vi "HelloWorld.vi"   [LabVIEW 2026]
uses:
  SDL3/Video/WindowFlags--ring.ctl
  SDL3/Pixels/PixelFormat--enum.ctl
  SDL3/Render/TextureAccess-enum.ctl
  SDL3/Init/InitFlags--ring.ctl
  SDL3/Events/MouseMotionEvent--cluster.ctl
  SDL3/Video/WindowID--integer.ctl
  SDL3/Mouse/MouseID--integer.ctl
  SDL3/Mouse/MouseButtonFlags--ring.ctl
  SDL3/Rect/FRect--cluster.ctl
  SDL3/Error/GetError-UiThread.vi
  SDL3/Error/GetError-AnyThread.vi
  SDL3/Pixels/PixelFormatEnumToU32.vi
  SDL3/LV-Utilities/IsNULL.vi
  SDL3/Pixels/U32ToPixelFormatEnum.vi
  <vilib>/Utility/error.llb/Error Cluster From Error Code.vi
  SDL3/Init/Init.lvlib
  SDL3/Video/Video.lvlib
  SDL3/Render/Render.lvlib
  SDL3/Pixels/Pixels.lvlib
  SDL3/Timer/Timer.lvlib
  SDL3/Events/Events.lvlib
  SDL3/Mouse/Mouse.lvlib
  SDL3/TTF/TTF.lvlib
  SDL3/Surface/Surface.lvlib
  SDL3/Rect/Rect.lvlib
types:
  T1 = enum32{"Invalid", "Standard", "Closed", "Hidden", "Minimized", "Maximized"}
  T2 = typedef "SDL3.lvlib/Events.lvlib/MouseMotionEvent--cluster.ctl" = cluster{"Timestamp":u64, "Window ID":T3, "Which":T4, "State":T5, "x":sgl, "y":sgl, "x Rel":sgl, "y Rel":sgl}
  T3 = typedef "SDL3.lvlib/Video.lvlib/WindowID--integer.ctl" = u32
  T4 = typedef "SDL3.lvlib/Mouse.lvlib/MouseID--integer.ctl" = u32
  T5 = typedef "SDL3.lvlib/Mouse.lvlib/MouseButtonFlags--ring.ctl" = u32
  T6 = typedef "SDL3.lvlib/Init.lvlib/InitFlags--ring.ctl" = u32
  T7 = typedef "SDL3.lvlib/Render.lvlib/TextureAccess-enum.ctl" = enum32{"SDL_TEXTUREACCESS_STATIC", "SDL_TEXTUREACCESS_STREAMING", "SDL_TEXTUREACCESS_TARGET"}
  T8 = typedef "SDL3.lvlib/Pixels.lvlib/PixelFormat--enum.ctl" = enum32{"SDL_PIXELFORMAT_UNKNOWN", "SDL_PIXELFORMAT_INDEX1LSB", "SDL_PIXELFORMAT_INDEX1MSB", "SDL_PIXELFORMAT_INDEX2LSB", "SDL_PIXELFORMAT_INDEX2MSB", "SDL_PIXELFORMAT_INDEX4LSB", "SDL_PIXELFORMAT_INDEX4MSB", "SDL_PIXELFORMAT_INDEX8", "SDL_PIXELFORMAT_RGB332", "SDL_PIXELFORMAT_XRGB4444", "SDL_PIXELFORMAT_XBGR4444", "SDL_PIXELFORMAT_XRGB1555", "SDL_PIXELFORMAT_XBGR1555", "SDL_PIXELFORMAT_ARGB4444", "SDL_PIXELFORMAT_RGBA4444", "SDL_PIXELFORMAT_ABGR4444", "SDL_PIXELFORMAT_BGRA4444", "SDL_PIXELFORMAT_ARGB1555", "SDL_PIXELFORMAT_RGBA5551", "SDL_PIXELFORMAT_ABGR1555", "SDL_PIXELFORMAT_BGRA5551", "SDL_PIXELFORMAT_RGB565", "SDL_PIXELFORMAT_BGR565", "SDL_PIXELFORMAT_RGB24", "SDL_PIXELFORMAT_BGR24", "SDL_PIXELFORMAT_XRGB8888", "SDL_PIXELFORMAT_RGBX8888", "SDL_PIXELFORMAT_XBGR8888", "SDL_PIXELFORMAT_BGRX8888", "SDL_PIXELFORMAT_ARGB8888", "SDL_PIXELFORMAT_RGBA8888", "SDL_PIXELFORMAT_ABGR8888", "SDL_PIXELFORMAT_BGRA8888", "SDL_PIXELFORMAT_XRGB2101010", "SDL_PIXELFORMAT_XBGR2101010", "SDL_PIXELFORMAT_ARGB2101010", "SDL_PIXELFORMAT_ABGR2101010", "SDL_PIXELFORMAT_RGB48", "SDL_PIXELFORMAT_BGR48", "SDL_PIXELFORMAT_RGBA64", "SDL_PIXELFORMAT_ARGB64", "SDL_PIXELFORMAT_BGRA64", "SDL_PIXELFORMAT_ABGR64", "SDL_PIXELFORMAT_RGB48_FLOAT", "SDL_PIXELFORMAT_BGR48_FLOAT", "SDL_PIXELFORMAT_RGBA64_FLOAT", "SDL_PIXELFORMAT_ARGB64_FLOAT", "SDL_PIXELFORMAT_BGRA64_FLOAT", "SDL_PIXELFORMAT_ABGR64_FLOAT", "SDL_PIXELFORMAT_RGB96_FLOAT", "SDL_PIXELFORMAT_BGR96_FLOAT", "SDL_PIXELFORMAT_RGBA128_FLOAT", "SDL_PIXELFORMAT_ARGB128_FLOAT", "SDL_PIXELFORMAT_BGRA128_FLOAT", "SDL_PIXELFORMAT_ABGR128_FLOAT", "SDL_PIXELFORMAT_YV12", "SDL_PIXELFORMAT_IYUV", "SDL_PIXELFORMAT_YUY2", "SDL_PIXELFORMAT_UYVY", "SDL_PIXELFORMAT_YVYU", "SDL_PIXELFORMAT_NV12", "SDL_PIXELFORMAT_NV21", "SDL_PIXELFORMAT_P010", "SDL_PIXELFORMAT_EXTERNAL_OES"}
  T9 = typedef "SDL3.lvlib/Video.lvlib/WindowFlags--ring.ctl" = u64
  T10 = typedef "SDL3.lvlib/Rect.lvlib/FRect--cluster.ctl" = cluster{"x":sgl, "y":sgl, "w":sgl, "h":sgl}
  T11 = typedef "SDL3.lvlib/Events.lvlib/EventType--enum.ctl" = enum16{"LV_NONE", "LV_UNSUPPORTED", "SDL_EVENT_QUIT", "SDL_EVENT_LOCALE_CHANGED", "SDL_EVENT_SYSTEM_THEME_CHANGED", "SDL_EVENT_DISPLAY_ORIENTATION", "SDL_EVENT_DISPLAY_ADDED", "SDL_EVENT_DISPLAY_REMOVED", "SDL_EVENT_DISPLAY_MOVED", "SDL_EVENT_DISPLAY_DESKTOP_MODE_CHANGED", "SDL_EVENT_DISPLAY_CURRENT_MODE_CHANGED", "SDL_EVENT_DISPLAY_CONTENT_SCALE_CHANGED", "SDL_EVENT_WINDOW_SHOWN", "SDL_EVENT_WINDOW_HIDDEN", "SDL_EVENT_WINDOW_EXPOSED", "SDL_EVENT_WINDOW_MOVED", "SDL_EVENT_WINDOW_RESIZED", "SDL_EVENT_WINDOW_PIXEL_SIZE_CHANGED", "SDL_EVENT_WINDOW_METAL_VIEW_RESIZED", "SDL_EVENT_WINDOW_MINIMIZED", "SDL_EVENT_WINDOW_MAXIMIZED", "SDL_EVENT_WINDOW_RESTORED", "SDL_EVENT_WINDOW_MOUSE_ENTER", "SDL_EVENT_WINDOW_MOUSE_LEAVE", "SDL_EVENT_WINDOW_FOCUS_GAINED", "SDL_EVENT_WINDOW_FOCUS_LOST", "SDL_EVENT_WINDOW_CLOSE_REQUESTED", "SDL_EVENT_WINDOW_HIT_TEST", "SDL_EVENT_WINDOW_ICCPROF_CHANGED", "SDL_EVENT_WINDOW_DISPLAY_CHANGED", "SDL_EVENT_WINDOW_DISPLAY_SCALE_CHANGED", "SDL_EVENT_WINDOW_SAFE_AREA_CHANGED", "SDL_EVENT_WINDOW_OCCLUDED", "SDL_EVENT_WINDOW_ENTER_FULLSCREEN", "SDL_EVENT_WINDOW_LEAVE_FULLSCREEN", "SDL_EVENT_WINDOW_DESTROYED", "SDL_EVENT_WINDOW_HDR_STATE_CHANGED", "SDL_EVENT_KEY_DOWN", "SDL_EVENT_KEY_UP", "SDL_EVENT_TEXT_EDITING", "SDL_EVENT_TEXT_INPUT", "SDL_EVENT_KEYMAP_CHANGED", "SDL_EVENT_KEYBOARD_ADDED", "SDL_EVENT_KEYBOARD_REMOVED", "SDL_EVENT_TEXT_EDITING_CANDIDATES", "SDL_EVENT_MOUSE_MOTION", "SDL_EVENT_MOUSE_BUTTON_DOWN", "SDL_EVENT_MOUSE_BUTTON_UP", "SDL_EVENT_MOUSE_WHEEL", "SDL_EVENT_MOUSE_ADDED", "SDL_EVENT_MOUSE_REMOVED", "SDL_EVENT_JOYSTICK_AXIS_MOTION", "SDL_EVENT_JOYSTICK_BALL_MOTION", "SDL_EVENT_JOYSTICK_HAT_MOTION", "SDL_EVENT_JOYSTICK_BUTTON_DOWN", "SDL_EVENT_JOYSTICK_BUTTON_UP", "SDL_EVENT_JOYSTICK_ADDED", "SDL_EVENT_JOYSTICK_REMOVED", "SDL_EVENT_JOYSTICK_BATTERY_UPDATED", "SDL_EVENT_JOYSTICK_UPDATE_COMPLETE", "SDL_EVENT_GAMEPAD_AXIS_MOTION", "SDL_EVENT_GAMEPAD_BUTTON_DOWN", "SDL_EVENT_GAMEPAD_BUTTON_UP", "SDL_EVENT_GAMEPAD_ADDED", "SDL_EVENT_GAMEPAD_REMOVED", "SDL_EVENT_GAMEPAD_REMAPPED", "SDL_EVENT_GAMEPAD_TOUCHPAD_DOWN", "SDL_EVENT_GAMEPAD_TOUCHPAD_MOTION", "SDL_EVENT_GAMEPAD_TOUCHPAD_UP", "SDL_EVENT_GAMEPAD_SENSOR_UPDATE", "SDL_EVENT_GAMEPAD_UPDATE_COMPLETE", "SDL_EVENT_GAMEPAD_STEAM_HANDLE_UPDATED", "SDL_EVENT_FINGER_DOWN", "SDL_EVENT_FINGER_UP", "SDL_EVENT_FINGER_MOTION", "SDL_EVENT_CLIPBOARD_UPDATE", "SDL_EVENT_DROP_FILE", "SDL_EVENT_DROP_TEXT", "SDL_EVENT_DROP_BEGIN", "SDL_EVENT_DROP_COMPLETE", "SDL_EVENT_DROP_POSITION", "SDL_EVENT_AUDIO_DEVICE_ADDED", "SDL_EVENT_AUDIO_DEVICE_REMOVED", "SDL_EVENT_AUDIO_DEVICE_FORMAT_CHANGED", "SDL_EVENT_SENSOR_UPDATE", "SDL_EVENT_PEN_PROXIMITY_IN", "SDL_EVENT_PEN_PROXIMITY_OUT", "SDL_EVENT_PEN_DOWN", "SDL_EVENT_PEN_UP", "SDL_EVENT_PEN_BUTTON_DOWN", "SDL_EVENT_PEN_BUTTON_UP", "SDL_EVENT_PEN_MOTION", "SDL_EVENT_PEN_AXIS", "SDL_EVENT_CAMERA_DEVICE_ADDED", "SDL_EVENT_CAMERA_DEVICE_REMOVED", "SDL_EVENT_CAMERA_DEVICE_APPROVED", "SDL_EVENT_CAMERA_DEVICE_DENIED", "SDL_EVENT_RENDER_TARGETS_RESET", "SDL_EVENT_RENDER_DEVICE_RESET", "SDL_EVENT_POLL_SENTINEL", "SDL_EVENT_USER"}
  T12 = typedef "SDL3.lvlib/Surface.lvlib/SurfaceFlags--ring.ctl" = u32
  T13 = cluster{"flag":T12, "format":T8, "w":i32, "h":i32, "pitch":i32}
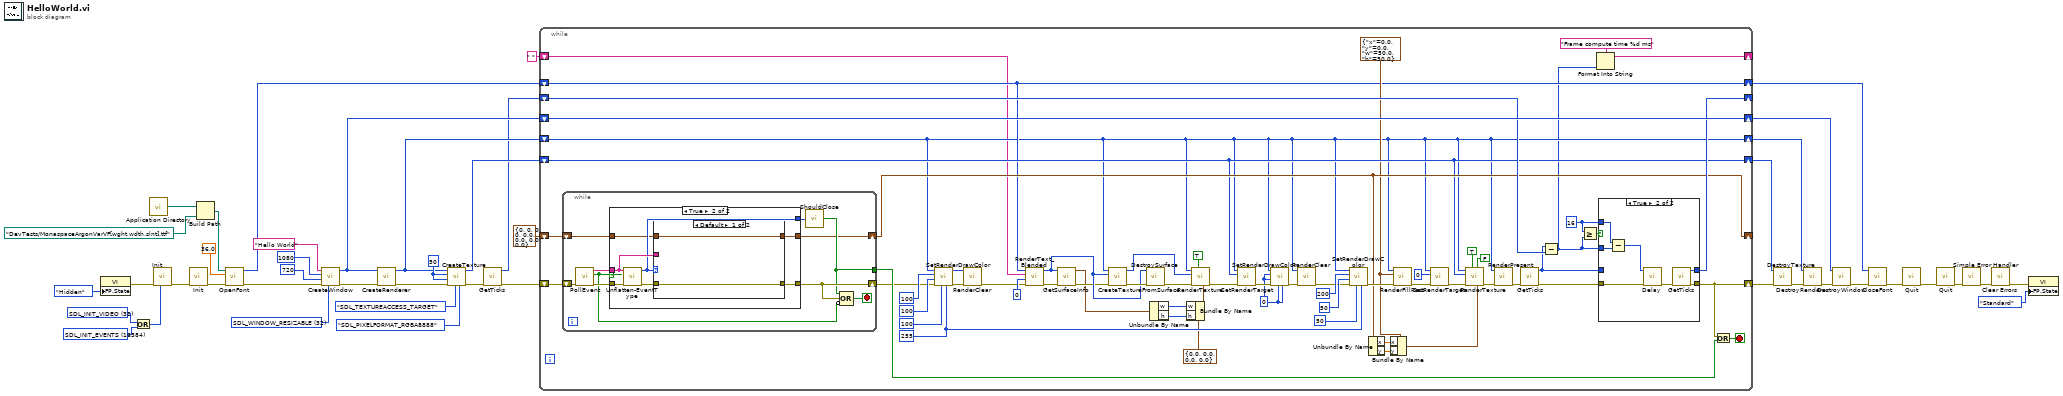
[diagram p0: block diagram]
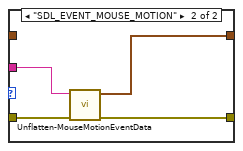
[diagram p3: hidden frame]
diagram:
  w16 = T6 16384 items=["NONE"=0, "SDL_INIT_AUDIO"=16, "SDL_INIT_VIDEO"=32, "SDL_INIT_JOYSTICK"=512, "SDL_INIT_HAPTIC"=4096, "SDL_INIT_GAMEPAD"=8192, "SDL_INIT_EVENTS"=16384, "SDL_INIT_SENSOR"=32768, "SDL_INIT_CAMER"=65536] ("y")
  w21 = T6 32 items=["NONE"=0, "SDL_INIT_AUDIO"=16, "SDL_INIT_VIDEO"=32, "SDL_INIT_JOYSTICK"=512, "SDL_INIT_HAPTIC"=4096, "SDL_INIT_GAMEPAD"=8192, "SDL_INIT_EVENTS"=16384, "SDL_INIT_SENSOR"=32768, "SDL_INIT_CAMER"=65536] ("InitFlags")
  w38 = 50 ("w")
  w43 = T9 32 items=["0"=0, "SDL_WINDOW_FULLSCREEN"=1, "SDL_WINDOW_OPENGL"=2, "SDL_WINDOW_OCCLUDED"=4, "SDL_WINDOW_HIDDEN"=8, "SDL_WINDOW_BORDERLESS"=16, "SDL_WINDOW_RESIZABLE"=32, "SDL_WINDOW_MINIMIZED"=64, "SDL_WINDOW_MAXIMIZED"=128, "SDL_WINDOW_MOUSE_GRABBED"=256, "SDL_WINDOW_INPUT_FOCUS"=512, "SDL_WINDOW_MOUSE_FOCUS"=1024, "SDL_WINDOW_EXTERNAL"=2048, "SDL_WINDOW_MODAL"=4096, "SDL_WINDOW_HIGH_PIXEL_DENSITY"=8192, "SDL_WINDOW_MOUSE_CAPTURE"=16384, "SDL_WINDOW_MOUSE_RELATIVE_MODE"=32768, "SDL_WINDOW_ALWAYS_ON_TOP"=65536, "SDL_WINDOW_UTILITY"=131072, "SDL_WINDOW_TOOLTIP"=262144, "SDL_WINDOW_POPUP_MENU"=524288, "SDL_WINDOW_KEYBOARD_GRABBED"=1048576, "SDL_WINDOW_VULKAN"=268435456, "SDL_WINDOW_METAL"=536870912, "SDL_WINDOW_TRANSPARENT"=1073741824, "SDL_WINDOW_NOT_FOCUSABLE"=2147483648] ("flags (0)")
  n1 = property class="VI"("FP.State"=T1."Hidden" ("Front Panel Window:State")) -> (error out=w26:errorcluster)  [unwired: 2 in, 1 out]
  n2 = Or(x=w21, y=w16) -> (x .or. y?=w17:T6)
  n3 = call <vilib>:"Application Directory.vi"() -> ("Application Directory"=w3:path)
  n4 = call "Init.vi"("InitFlags"=w17, "No Error"=w26) -> ("error out"=w13:errorcluster)  [unwired: 9 in]
  n5 = call "Init.vi"("No Error"=w13) -> ("error out"=w11:errorcluster)  [unwired: 10 in]
  n6 = Build Path(base path=w3, name or relative path=path "DevTests/MonaspaceArgonVarVF[wght,wdth,slnt].ttf") -> (appended path=w4:path)
  n7 = call "OpenFont.vi"("No Error"=w11, "Pt Size"=sgl 36.0, "File"=w4) -> ("error out"=w10:errorcluster, "Font [TTF_Font *]"=w7:i64)  [unwired: 7 in]
  n8 = call "CreateWindow.vi"("Flags (0)"=w43, "No Error"=w10, "h"=720, "w"=1080, "Title"="Hello World" ("title")) -> ("Error Out"=w42:errorcluster, "Window [SDL_Window *]"=w34:i64)  [unwired: 5 in]
  n9 = call "CreateRenderer.vi"("No Error"=w42, "Window [SDL_Window *]"=w34) -> ("Error Out"=w39:errorcluster, "Renderer [SDL_Renderer *]"=w33:i64)  [unwired: 8 in]
  n10 = call "CreateTexture.vi"("Pixel Format"=PixelFormat--enum."SDL_PIXELFORMAT_RGBA8888" ("pixel_format"), "Texture Access"=TextureAccess-enum."SDL_TEXTUREACCESS_TARGET" ("texture_access"), "No Error"=w39, "h"=w38, "w"=w38, "Renderer [SDL_Renderer *]"=w33) -> ("error out"=w20:errorcluster, "Texture [SDL_Texture *]"=w32:i64)  [unwired: 4 in]
  n11 = call "GetTicks.vi"("No Error"=w20) -> ("error out"=w19:errorcluster, "Ticks [ms]"=w18:u64)  [unwired: 9 in]
  n12 = while {
    shift-right: [w77] -> w29
    shift-left: w32 -> [w77]
    shift-right: [w60] -> w30
    shift-left: w33 -> [w60]
    shift-right: [w104] -> w31
    shift-left: w34 -> [w104]
    shift-right: [w67] -> w41
    shift-left: w19 -> [w82]
    shift-right: [w89] -> _
    shift-left: w18 -> [w86]
    shift-right: [w80] -> _
    shift-left: T2 {"Timestamp"=0, "Window ID"=0, "Which"=0, "State"=0, "x"=0.0, "y"=0.0, "x Rel"=0.0, "y Rel"=0.0} ("MouseMotionEvent") -> [w81]
    shift-right: [w65] -> w6
    shift-left: w7 -> [w65]
    shift-right: [w46] -> _
    shift-left: " " -> [w48]
    stop <- w68 stop-if-true
    w72 = u8 0 ("r")
    w85 = u64 16
    w70 = cluster{"x":sgl, "y":sgl, "w":sgl, "h":sgl} {"x"=0.0, "y"=0.0, "w"=50.0, "h"=50.0} ("rect")
    w74 = u8 255 ("a")
    n13 = while {
      shift-right: [w109] -> w62
      shift-left: w82 -> [w114]
      tunnel: [w107] -> w69
      shift-right: [w106] -> w80
      shift-left: w81 -> [w105]
      stop <- w113 stop-if-true
      n14 = call "PollEvent.vi"("No Error"=w114) -> ("error out"=w112:errorcluster, "Event Occured?"=w110:bool, "Event Binary Data"=w111:string)  [unwired: 8 in]
      n15 = case shown="True" w110 {
        tunnel: w112 -> [w116 w123]
        tunnel: w111 -> [_ w122]
        tunnel: [w116 w119] -> w109
        tunnel: [_ w121] -> w108
        tunnel: [w115 w118] -> w106
        tunnel: w105 -> [w115 w117]
        frame False {
        }
        frame True {
          n16 = call "Unflatten-EventType.vi"("error in (no error)"=w123, "Event Binary Data In"=w122) -> ("error out"=w120:errorcluster, "EventType"=w121:T11)  [unwired: 8 in]
          n17 = case shown="Default" w121 {
            tunnel: w122 -> [_ w128]
            tunnel: w120 -> [w125 w129]
            tunnel: [w125 w127] -> w119
            tunnel: [w124 w126] -> w118
            tunnel: w117 -> [w124 _]
            frame Default {
            }
            frame "SDL_EVENT_MOUSE_MOTION" {
              n18 = call "Unflatten-MouseMotionEventData.vi"("error in (no error)"=w129, "Event Binary Data"=w128) -> ("error out"=w127:errorcluster, "MouseMotionEvent"=w126:T2)  [unwired: 8 in]
            }
          }
        }
      }
      n19 = call "ShouldClose.vi"("EventType"=w108) -> ("Close?"=w107:bool)
      n20 = Compound Arithmetic op=OR(w107, w109, invert w110) -> (w113:bool)
    }
    n21 = call "SetRenderDrawColor.vi"("a"=w74, "b"=u8 100, "No Error"=w62, "g"=u8 100, "r"=u8 100, "Renderer [SDL_Renderer *]"=w60) -> ("error out"=w101:errorcluster)  [unwired: 5 in]
    n22 = call "RenderClear.vi"("No Error"=w101, "Renderer [SDL_Renderer *]"=w60) -> ("error out"=w63:errorcluster)  [unwired: 9 in]
    n23 = call "RenderText_Blended.vi"("No Error"=w63, "FG Color"=u32 0, "Text"=w48, "Font [TTF_Font *]"=w65) -> ("error out"=w55:errorcluster, "Surface [SDL_Surface *]"=w54:i64)  [unwired: 6 in]
    n24 = call "GetSurfaceInfo.vi"("No Error"=w55, "Surface [SDL_Surface *]"=w54) -> ("error out"=w53:errorcluster, "Surface Info"=w51:T13)  [unwired: 8 in]
    n25 = call "CreateTextureFromSurface.vi"("No Error"=w53, "Surface [SDL_Surface *]"=w54, "Renderer [SDL_Renderer *]"=w60) -> ("error out"=w64:errorcluster, "Texture [SDL_Texture *]"=w59:i64)  [unwired: 7 in]
    n26 = call "DestroySurface.vi"("No Error"=w64, "Surface [SDL_Surface *]"=w54) -> ("error out"=w61:errorcluster)  [unwired: 9 in]
    n27 = Unbundle By Name(w51) -> ("w"=w50:i32, "h"=w49:i32)
    n28 = Bundle By Name(cluster=T10 {"x"=0.0, "y"=0.0, "w"=0.0, "h"=0.0} ("Dstrect"), "w"=w50, "h"=w49) -> (w52:T10)
    n29 = call "RenderTexture.vi"("Dstrect"=w52, "Entire Texture (F)"=TRUE, "No Error"=w61, "Texture [SDL_Texture *]"=w59, "Renderer [SDL_Renderer *]"=w60) -> ("error out"=w58:errorcluster)  [unwired: 6 in]
    n30 = call "SetRenderTarget.vi"("No Error"=w58, "Texture [SDL_Texture *]"=w77, "Renderer [SDL_Renderer *]"=w60) -> ("error out"=w76:errorcluster)  [unwired: 8 in]
    n31 = call "SetRenderDrawColor.vi"("a"=w72, "b"=w72, "No Error"=w76, "g"=w72, "r"=w72, "Renderer [SDL_Renderer *]"=w60) -> ("error out"=w75:errorcluster)  [unwired: 5 in]
    n32 = call "RenderClear.vi"("No Error"=w75, "Renderer [SDL_Renderer *]"=w60) -> ("error out"=w73:errorcluster)  [unwired: 9 in]
    n33 = call "SetRenderDrawColor.vi"("a"=w74, "b"=u8 50, "No Error"=w73, "g"=u8 50, "r"=u8 200, "Renderer [SDL_Renderer *]"=w60) -> ("error out"=w94:errorcluster)  [unwired: 5 in]
    n34 = Unbundle By Name(w80) -> ("x"=w79:sgl, "y"=w78:sgl)
    n35 = Bundle By Name(cluster=w70, "x"=w79, "y"=w78) -> (w71:cluster{"x":sgl, "y":sgl, "w":sgl, "h":sgl})
    n36 = call "RenderFillRect.vi"("No Error"=w94, "Rect"=w70, "Renderer [SDL_Renderer *]"=w60) -> ("error out"=w90:errorcluster)  [unwired: 8 in]
    n37 = call "SetRenderTarget.vi"("No Error"=w90, "Texture [SDL_Texture *]"=i64 0 ("texture [SDL_Texture *]"), "Renderer [SDL_Renderer *]"=w60) -> ("error out"=w102:errorcluster)  [unwired: 8 in]
    n38 = call "RenderTexture.vi"("Dstrect"=w71, "Entire Rendering Target (F)"=FALSE, "Entire Texture (F)"=TRUE, "No Error"=w102, "Texture [SDL_Texture *]"=w77, "Renderer [SDL_Renderer *]"=w60) -> ("error out"=w103:errorcluster)  [unwired: 5 in]
    n39 = call "RenderPresent.vi"("No Error"=w103, "Renderer [SDL_Renderer *]"=w60) -> ("error out"=w88:errorcluster)  [unwired: 9 in]
    n40 = call "GetTicks.vi"("No Error"=w88) -> ("error out"=w87:errorcluster, "Ticks [ms]"=w83:u64)  [unwired: 9 in]
    n41 = Subtract(x=w83, y=w86) -> (x-y=w47:u64)
    n42 = Greater Or Equal?(x=w85, y=w47) -> (x >= y?=w84:bool)
    n43 = Format Into String(format string="Frame compute time %d ms", w47) -> (resulting string=w46:string)  [unwired: 2 in, 1 out]
    n44 = case shown="True" w84 {
      tunnel: [w130 w138] -> w67
      tunnel: [w131 w137] -> w89
      tunnel: w87 -> [w130 w136]
      tunnel: w85 -> [_ w135]
      tunnel: w47 -> [_ w134]
      tunnel: w83 -> [w131 _]
      frame False {
      }
      frame True {
        n45 = Subtract(x=w135, y=w134) -> (x-y=w132:u64)
        n46 = call "Delay.vi"("No Error"=w136, "ms"=w132) -> ("error out"=w133:errorcluster)  [unwired: 9 in]
        n47 = call "GetTicks.vi"("No Error"=w133) -> ("error out"=w138:errorcluster, "Ticks [ms]"=w137:u64)  [unwired: 9 in]
      }
    }
    n48 = Or(x=w67, y=w69) -> (x .or. y?=w68:bool)
  }
  n49 = call "DestroyTexture.vi"("No Error"=w41, "Texture [SDL_Texture *]"=w29) -> ("error out"=w35:errorcluster)  [unwired: 9 in]
  n50 = call "DestroyRenderer.vi"("No Error"=w35, "Rrenderer [SDL_Renderer *]"=w30) -> ("error out"=w40:errorcluster)  [unwired: 9 in]
  n51 = call "DestroyWindow.vi"("No Error"=w40, "Window [SDL_Window*]"=w31) -> ("Error Out"=w9:errorcluster)  [unwired: 9 in]
  n52 = call "CloseFont.vi"("No Error"=w9, "Font [TTF_Font *]"=w6) -> ("error out"=w8:errorcluster)  [unwired: 9 in]
  n53 = call "Quit.vi"("No Error"=w8) -> ("error out"=w12:errorcluster)  [unwired: 10 in]
  n54 = call "Quit.vi"("No Error"=w12) -> ("error out"=w24:errorcluster)  [unwired: 10 in]
  n55 = call <vilib>:"Simple Error Handler.vi"("error in (no error)"=w24) -> ("error out"=w23:errorcluster)  [unwired: 4 in, 4 out]
  n56 = call <vilib>:"Clear Errors.vi"("error in (no error)"=w23) -> ("error out"=w22:errorcluster)  [unwired: 5 in, 1 out]
  n57 = property class="VI"(error in=w22, "FP.State"=T1."Standard" ("Front Panel Window:State")) -> ()  [unwired: 1 in, 2 out]
